vi "Configure Temperature.vi"   [LabVIEW 2022 SP3, in "Agilent 34401.lvlib"]
doc: "Configures the settings for 2-wire and 4-wire RTD and Thermistor probe types. \n\n<B>Note:</B>\n\nThis VI only applies to the 34410/34411 models."
uses:
  <instrlib>/Agilent 34401/Agilent 34401.lvlib
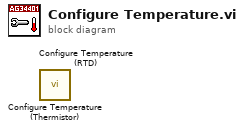
[diagram p0: block diagram]
diagram:
  n1 = call <instrlib>:"Configure Temperature (Thermistor).vi"() -> ()  [unwired: 14 in, 2 out]
  n2 = call <instrlib>:"Configure Temperature (RTD).vi"() -> ()  [unwired: 14 in, 2 out]
